vi "slink set scale.vi"(6 "ChannelEnable":cluster{"Channel 1":T2, "Channel 2":T2}, 7 "Numeric":i32, 9 "Simulation":T2, 10 "Scale":T1, 11 "VISA Refnum in":refnum<visa-resource-name>) -> ()   [LabVIEW 2020, in "Gentec SlinkUSB.lvclass"]
uses:
  Gentec SlinkUSB.lvclass
  OnOffTypeDef.ctl
  sclae_typdef.ctl
  Serial Commands Slink.ctl
panel:
  out "error out":errorcluster
  in  "error in (no error)":errorcluster
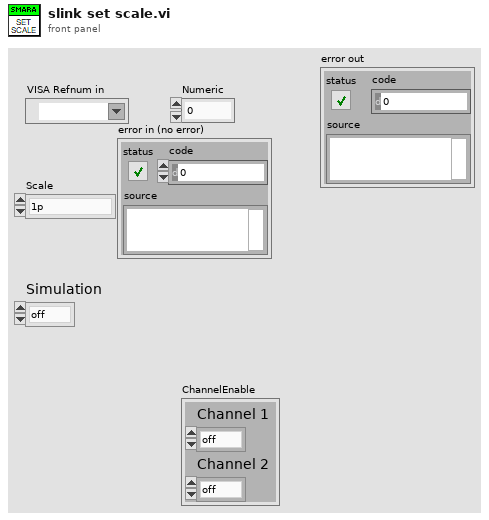
[diagram p1: front panel]
types:
  T1 = typedef "sclae_typdef.ctl" = enum16{"1p", "3p", "10p", "30p", "100p", "300p", "1n", "3n", "10n", "30n", "100n", "300n", "1u", "3u", "10u", "30u", "100u", "300u", "1m", "3m", "10m", "30m", "100m", "300m", "1", "3", "10", "30", "100", "300", "1k", "3k", "10k", "30k", "100k", "300k", "1meg", "3meg", "10meg", "30meg", "100meg", "300meg"}
  T2 = typedef "OnOffTypeDef.ctl" = enum16{"off", "on"}
  T3 = typedef "Serial Commands Slink.ctl" = i32
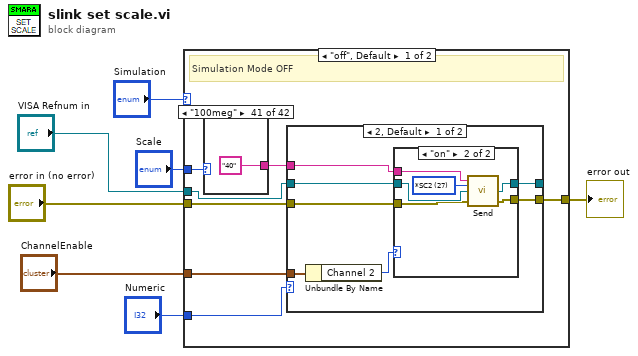
[diagram p0: block diagram]
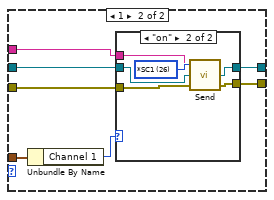
[diagram p3: hidden frame]
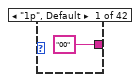
[diagram p5: hidden frame]
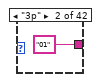
[diagram p6: hidden frame]
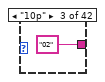
[diagram p7: hidden frame]
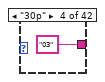
[diagram p8: hidden frame]
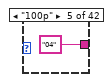
[diagram p9: hidden frame]
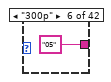
[diagram p10: hidden frame]
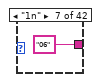
[diagram p11: hidden frame]
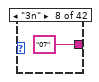
[diagram p12: hidden frame]
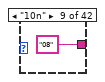
[diagram p13: hidden frame]
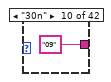
[diagram p14: hidden frame]
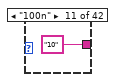
[diagram p15: hidden frame]
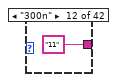
[diagram p16: hidden frame]
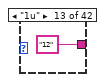
[diagram p17: hidden frame]
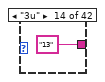
[diagram p18: hidden frame]
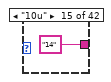
[diagram p19: hidden frame]
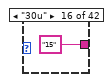
[diagram p20: hidden frame]
diagram:
  n1 = case shown="\"off\", Default" "Simulation" {
    tunnel: "Scale" -> [w14 _]
    tunnel: "Numeric" -> [w13 _]
    tunnel: "VISA Refnum in" -> [w12 _]
    tunnel: "ChannelEnable" -> [w10 _]
    tunnel: "error in (no error)" -> [w9 w87]
    tunnel: [w8 w87] -> w1
    frame "off", Default {
      # "Simulation Mode OFF"
      n2 = case shown="\"100meg\"" w14 {
        tunnel: ["00" "01" "02" "03" "04" "05" "06" "07" "08" "09" "10" "11" "12" "13" "14" "15" "16" "17" "18" "19" "20" "21" "22" "23" "24" "25" "26" "27" "28" "29" "30" "31" "32" "33" "34" "35" "36" "37" "38" "39" "40" "41"] -> w11
        frame "1p", Default {
        }
        frame "3p" {
        }
        frame "10p" {
        }
        frame "30p" {
        }
        frame "100p" {
        }
        frame "300p" {
        }
        frame "1n" {
        }
        frame "3n" {
        }
        frame "10n" {
        }
        frame "30n" {
        }
        frame "100n" {
        }
        frame "300n" {
        }
        frame "1u" {
        }
        frame "3u" {
        }
        frame "10u" {
        }
        frame "30u" {
        }
        frame "100u" {
        }
        frame "300u" {
        }
        frame "1m" {
        }
        frame "3m" {
        }
        frame "10m" {
        }
        frame "30m" {
        }
        frame "100m" {
        }
        frame "300m" {
        }
        frame "1" {
        }
        frame "3" {
        }
        frame "10" {
        }
        frame "30" {
        }
        frame "100" {
        }
        frame "300" {
        }
        frame "1k" {
        }
        frame "3k" {
        }
        frame "10k" {
        }
        frame "30k" {
        }
        frame "100k" {
        }
        frame "300k" {
        }
        frame "1meg" {
        }
        frame "3meg" {
        }
        frame "10meg" {
        }
        frame "30meg" {
        }
        frame "100meg" {
        }
        frame "300meg" {
        }
      }
      n3 = case shown="2, Default" w13 {
        tunnel: w11 -> [w21 w36]
        tunnel: w12 -> [w20 w35]
        tunnel: [w19 w34] -> _
        tunnel: w10 -> [w18 w33]
        tunnel: w9 -> [w16 w31]
        tunnel: [w15 w30] -> w8
        frame 2, Default {
          n4 = Unbundle By Name(w18) -> ("Channel 2"=w17:T2)
          n5 = case shown="\"on\"" w17 {
            tunnel: w21 -> [_ w28]
            tunnel: w20 -> [w23 w27]
            tunnel: [w23 w26] -> w19
            tunnel: w16 -> [w22 w25]
            tunnel: [w22 w24] -> w15
            frame "off", Default {
            }
            frame "on" {
              w29 = T3 27 items=["*RST", "*VER", "*CA1", "*CA2", "*SS100", "*SS200", "*SU1", "*SU2", "*SD1", "*SD2", "*CS1", "*CS2", "*AT1", "*AT2", "*AN1", "*AN2", "*PW1", "*PW2", "*TL1", "*TL2", "*ST1", "*ST2", "*ET1", "*ET2", "*EM1", "*EM2", "*SC1", "*SC2"] ("string to write")
              n6 = call "Send.vi"("string to write"=w29, "error in (no error)"=w25, "port number"=w27, "Option"=w28) -> ("error out"=w24:errorcluster, "VISA resource name out"=w26:refnum<visa-resource-name>)
            }
          }
        }
        frame 1 {
          n7 = Unbundle By Name(w33) -> ("Channel 1"=w32:T2)
          n8 = case shown="\"on\"" w32 {
            tunnel: w36 -> [_ w43]
            tunnel: w35 -> [w38 w42]
            tunnel: [w38 w41] -> w34
            tunnel: w31 -> [w37 w40]
            tunnel: [w37 w39] -> w30
            frame "off", Default {
            }
            frame "on" {
              w44 = T3 26 items=["*RST", "*VER", "*CA1", "*CA2", "*SS100", "*SS200", "*SU1", "*SU2", "*SD1", "*SD2", "*CS1", "*CS2", "*AT1", "*AT2", "*AN1", "*AN2", "*PW1", "*PW2", "*TL1", "*TL2", "*ST1", "*ST2", "*ET1", "*ET2", "*EM1", "*EM2", "*SC1", "*SC2"] ("string to write")
              n9 = call "Send.vi"("string to write"=w44, "error in (no error)"=w40, "port number"=w42, "Option"=w43) -> ("error out"=w39:errorcluster, "VISA resource name out"=w41:refnum<visa-resource-name>)
            }
          }
        }
      }
    }
    frame "on" {
      # "Simulation Mode ON"
    }
  }
  "error out" <- w1
